vi "NI VeriStand - Get Engine State.vi"(8 "error in (no error)":errorcluster, 11 "WorkspaceManager in":T2) -> (0 "error out":errorcluster, 1 "IP Address":string, 2 "System State":T1 items=["Idle", "Active"], 3 "WorkspaceManager  out":T2, 5 "System Definition File":path, 7 "Workspace File":path)   [LabVIEW 2020, in "NI_VS Workspace ExecutionAPI.lvlib"]
doc: "Returns information about the status of the VeriStand Engine, including the IP address of the execution host, names of the workspace and system definition files currently running, and whether the VeriStand Engine is idle or active."
uses:
  <vilib>/NI VeriStand/Execution/Workspace/NI_VS Workspace ExecutionAPI.lvlib
  <vilib>/NI VeriStand/Execution/Workspace/WorkspaceAPI.ctl
  NationalInstruments.VeriStand.ClientAPI
  <vilib>/NI VeriStand/Execution/Workspace/SystemState.ctl
panel:
  # "This VI has been deprecated in favor of NI VeriStand - Get System State.vi. If there are multiple targets in a System Definition, this function will only return the IP Address for the first target."
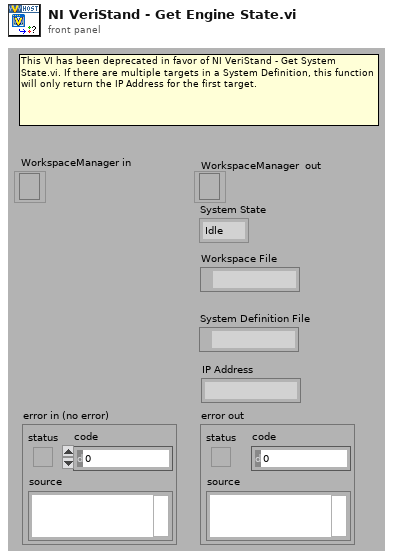
[diagram p1: front panel]
types:
  T1 = typedef "NI_VS Workspace ExecutionAPI.lvlib/SystemState.ctl" = u8
  T2 = typedef "NI_VS Workspace ExecutionAPI.lvlib/WorkspaceAPI.ctl" = refnum<k24>
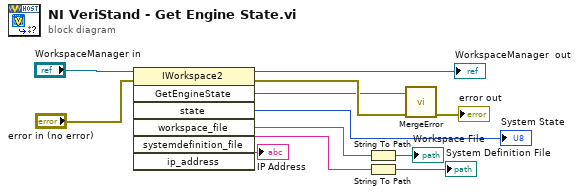
[diagram p0: block diagram]
diagram:
  n1 = invoke class="IWorkspace2" method="GetEngineState"(reference="WorkspaceManager in", error in="error in (no error)") -> (reference out=→"WorkspaceManager  out":T2, error out=w10:errorcluster, "GetEngineState"=w9:refnum<k24>, "state"=→"System State":u8, "workspace_file"=w5:string, "systemdefinition_file"=w2:string, "ip_address"=→"IP Address":string)  [unwired: 5 in]
  n2 = String To Path(string=w5) -> (path=→"Workspace File":path)
  n3 = String To Path(string=w2) -> (path=→"System Definition File":path)
  n4 = call <vilib>:"MergeError.vi"("error in (no error)"=w10, "Error"=w9) -> ("error out"=→"error out":errorcluster)  [unwired: 9 out]
